vi "Build dt Ramp.vi"(8 "error in (no error)":errorcluster, 9 "Stop idx":i32, 10 "Start idx (0)":i32, 11 "Frequency (Hz)":dbl) -> (0 "error out":errorcluster, 3 "Ramp (s)":dbl[](array[numeric]))   [LabVIEW 2016]
uses:
  <vilib>/Analysis/1siggen.llb/Ramp Pattern by Delta.vi
  <vilib>/Analysis/NI_AALBase.lvlib
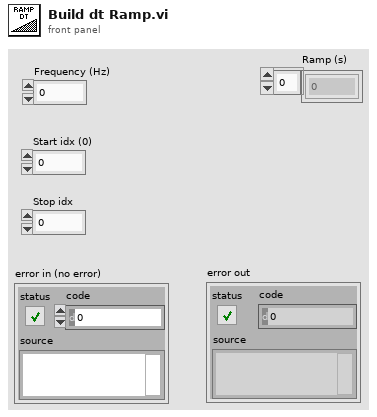
[diagram p1: front panel]
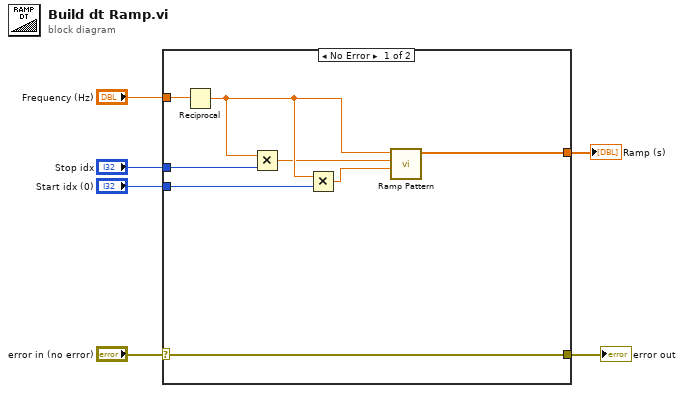
[diagram p0: block diagram]
diagram:
  n1 = case shown="No Error" "error in (no error)" {
    selector: "error in (no error)" -> [w14 w15]
    tunnel: [w14 w15] -> w5
    tunnel: "Start idx (0)" -> [w12 _]
    tunnel: "Stop idx" -> [w11 _]
    tunnel: "Frequency (Hz)" -> [w13 _]
    tunnel: [w7 _] -> w1
    frame No Error {
      n2 = Reciprocal(x=w13) -> (1/x=w10:dbl)
      n3 = Multiply(x=w10, y=w11) -> (x*y=w9:dbl)
      n4 = Multiply(x=w10, y=w12) -> (x*y=w8:dbl)
      n5 = call-poly <vilib>:"Ramp Pattern.vi"("start"=w8, "end"=w9, "delta"=w10) -> ("Ramp Pattern"=w7:dbl[])  [unwired: 6 in, 2 out]
    }
    frame Error {
    }
  }
  "error out" <- w5
  "Ramp (s)" <- w1
